vi "PH_ImageCalibrator.write Dark Pic.vi"(0 "i ref in":refnum<vi>, 2 "Cam Image":T1, 5 "error in (no error)":errorcluster) -> (14 "i ref out":refnum<vi>, 19 "error out":errorcluster)   [LabVIEW 2014, in "PH_ImageCalibrator.lvlib"]
doc: "This VI adds the incoming Cam Image to the background image and sets the number of accumulated pics up by one."
uses:
  PH_ImageCalibrator.lvlib
  <vilib>/vision/Image Controls.llb/IMAQ Image.ctl
  CS_Core/BaseSM/BaseSM.lvlib
  <vilib>/vision/NI_Vision_Development_Module.lvlib
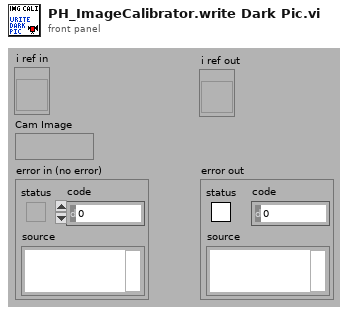
[diagram p1: front panel]
types:
  T1 = typedef "IMAQ Image.ctl" = refnum<image>
  T2 = typedef "PH_ImageCalibrator.lvlib/PH_ImageCalibrator.i attribute.ctl" = cluster{"GUI Refs":cluster{"Available Cams":refnum<vi>, "OK":refnum<vi>, "Skip":refnum<vi>, "Repeat":refnum<vi>, "Cancel":refnum<vi>, "Length [mm]":refnum<vi>, "Energy [mJ]":refnum<vi>, "Dialog":refnum<vi>}, "Cam instances":string[], "Dark Pics":cluster{"#":i32, "BI taken":bool}, "Lin Cali":cluster{"Distance [Pixel]":dbl, "Distance [mm]":dbl, "Lin Cali Factor [mm/Pixel]":dbl}, "Energy Cali":cluster{"Pixelsum":dbl, "Energy [mJ]":dbl, "Energy Cali factor [mJ/Pixelsum]":dbl, "Underground subtracted?":bool, "#":i32}, "Images":cluster{"Background":T1, "Energy":T1}}
  T3 = typedef "Image Type" = u32
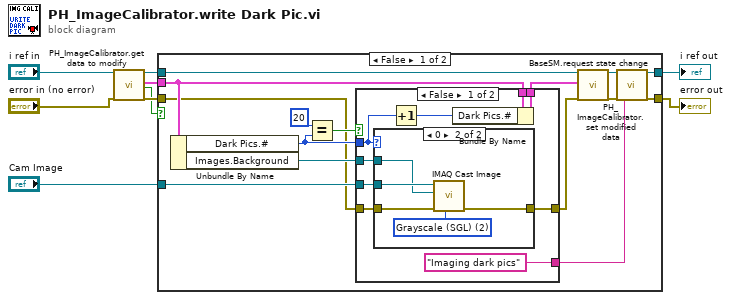
[diagram p0: block diagram]
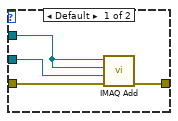
[diagram p2: hidden frame]
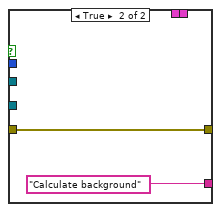
[diagram p3: hidden frame]
diagram:
  n1 = call "PH_ImageCalibrator.get data to modify.vi"("i ref in"="i ref in", "error in (no error)"="error in (no error)") -> ("i ref out"=w6:refnum<vi>, "i attribute"=w9:T2, "timed out"=w2:bool, "error out"=w3:errorcluster)  [unwired: 14 in]
  n2 = case shown="False" w2 {
    tunnel: "Cam Image" -> [w23 _]
    tunnel: w9 -> [w24 _]
    tunnel: [w19 w47] -> w8
    tunnel: w6 -> [w10 w47]
    tunnel: [w17 w46] -> w4
    tunnel: w3 -> [w11 w46]
    frame False {
      n3 = Unbundle By Name(w24) -> ("Dark Pics.#"=w22:i32, "Images.Background"=w13:T1)
      n4 = Equal?(x=20, y=w22) -> (x = y?=w21:bool)
      n5 = case shown="False" w21 {
        tunnel: w24 -> [w31 w43]
        tunnel: w23 -> [w33 _]
        tunnel: w22 -> [w29 _]
        tunnel: ["Imaging dark pics" "Calculate background"] -> w16
        tunnel: w13 -> [w28 _]
        tunnel: [w27 w44] -> w15
        tunnel: w11 -> [w26 w44]
        tunnel: [w25 w43] -> w14
        frame False {
          n6 = case shown="0" w29 {
            tunnel: w33 -> [w35 w42]
            tunnel: w28 -> [w34 w38]
            tunnel: [w36 w40] -> w27
            tunnel: w26 -> [w37 w39]
            frame Default {
              n7 = call "IMAQ Add"("Image Src A"=w34, "Image Dst"=w34, "Image Src B"=w35, "error in (no error)"=w37) -> ("error out"=w36:errorcluster)  [unwired: 3 in, 1 out]
            }
            frame 0 {
              w41 = T3 2 items=["Grayscale (U8)", "Grayscale (I16)", "Grayscale (SGL)", "Complex (CSG)", "RGB (U32)", "HSL (U32)", "RGB (U64)"] ("Image Type")
              n8 = call "IMAQ Cast Image"("Image Type"=w41, "error in (no error)"=w39, "Image Dst"=w38, "Image Src"=w42) -> ("error out"=w40:errorcluster)  [unwired: 6 in, 1 out]
            }
          }
          n9 = Increment(x=w29) -> (x+1=w30:i32)
          n10 = Bundle By Name(cluster=w31, "Dark Pics.#"=w30) -> (w25:T2)
        }
        frame True {
        }
      }
      n11 = call "PH_ImageCalibrator.set modified data.vi"("i ref in"=w10, "i attribute"=w14, "error in (no error)"=w15) -> ("i ref out"=w20:refnum<vi>, "error out"=w18:errorcluster)  [unwired: 15 in]
      n12 = call "BaseSM.request state change.vi"("i ref in"=w20, "error in (no error)"=w18, "requested state"=w16) -> ("i ref out"=w19:refnum<vi>, "error out"=w17:errorcluster)  [unwired: 13 in, 2 out]
    }
    frame True {
    }
  }
  "i ref out" <- w8
  "error out" <- w4
